vi "Read Command String.vi"(8 "error in":errorcluster, 11 "lia rt in":refnum<class "Lock-In Amplifier Example RT.lvclass">) -> (0 "error out":errorcluster, 1 "valid":bool, 2 "message":T1, 3 "lia rt out":refnum<class "Lock-In Amplifier Example RT.lvclass">)   [LabVIEW 2017, in "Lock-In Amplifier Example RT.lvclass"]
uses:
  Lock-In Amplifier Example RT.lvclass
  shared/Public/message.ctl
  Properties/Server_GET.vi
  server/RT FlexRIO Server TCP.lvclass
  shared/Lock-In Amplifier Example Shared.lvlib
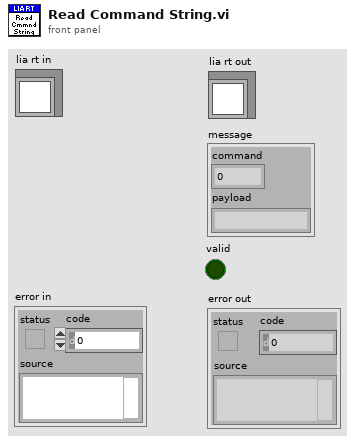
[diagram p1: front panel]
types:
  T1 = typedef "Lock-In Amplifier Example Shared.lvlib/message.ctl" = cluster{"command":u32, "payload":string}
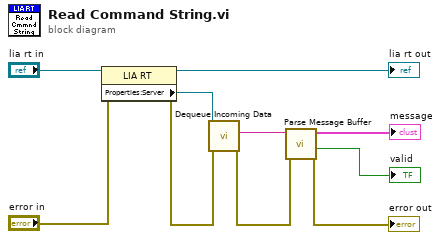
[diagram p0: block diagram]
diagram:
  n1 = property class="LIA RT"(reference="lia rt in", error in="error in") -> (reference out=→"lia rt out":refnum<class "Lock-In Amplifier Example RT.lvclass">, error out=w7:errorcluster, "Properties:Server"=w9:refnum<class "RT FlexRIO Server TCP.lvclass">)
  n2 = call "Dequeue Incoming Data.vi"("error in"=w7, "server in"=w9) -> ("error out"=w4:errorcluster, "string out"=w5:string)  [unwired: 7 in, 1 out]
  n3 = call "Parse Message Buffer.vi"("error in"=w4, "string in"=w5) -> ("error out"=→"error out":errorcluster, "valid"=→"valid":bool, "message"=→"message":T1)  [unwired: 7 in]
